vi "UpperSwitchPressed.vi"() -> ()   [LabVIEW 2017]
panel:
  out "SwitchPressedUp":bool
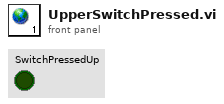
[diagram p1: front panel]
diagram:
